vi "SecondBlink.vi"() -> ()   [LabVIEW 2010]
panel:
  out "x = y?":bool
  out "double precision float":dbl format="%_20f"
  out "32bit integer":i64
  out "x-y*floor(x/y)":i32
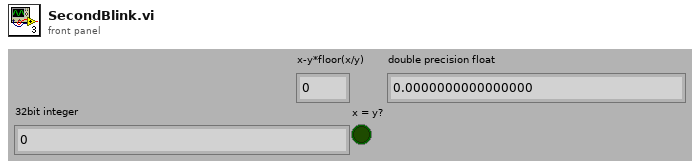
[diagram p1: front panel]
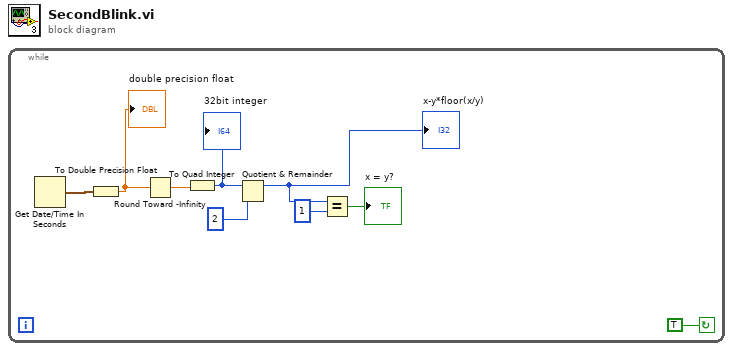
[diagram p0: block diagram]
diagram:
  n1 = while {
    stop <- TRUE continue-if-true
    n2 = Get Date/Time In Seconds() -> (seconds since 1Jan1904=w9:timestamp)
    n3 = To Double Precision Float(number=w9) -> (double precision float=w7:dbl)
    "double precision float" <- w7
    n4 = Round Toward -Infinity(1:w7) -> (0:w6:dbl)
    n5 = To Quad Integer(1:w6) -> (0:w5:i64)
    "32bit integer" <- w5
    n6 = Quotient & Remainder(x=w5, y=2) -> (x-y*floor(x/y)=w3:i64)  [unwired: 1 out]
    "x-y*floor(x/y)" <- w3
    n7 = Equal?(x=w3, y=i64 1) -> (x = y?=→"x = y?":bool)
  }
